vi "Shoot.vi"(10 "User Input":dbl, 11 "Numeric":dbl) -> ()   [LabVIEW 2012]
uses:
  Robot Global Data.vi
panel:
  # "Shoot"
  # "Shooter power ;1. Frount of the 3 point target\n                          2. Frount of 2 point target\n                          3. Key frount of 3 point target \n                          4. User Input"
  # "Input  0 to -1"
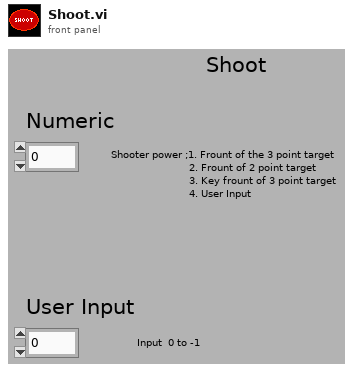
[diagram p1: front panel]
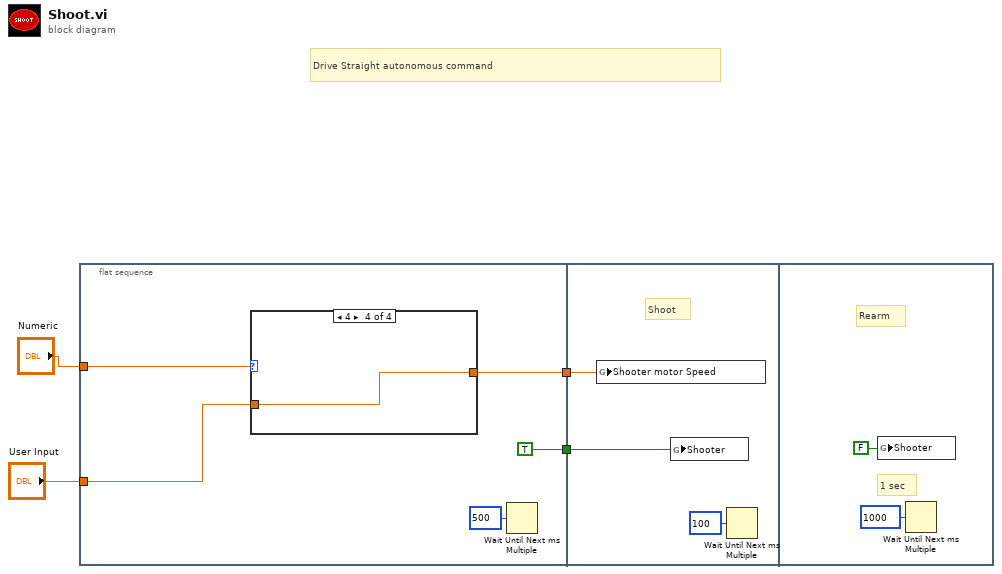
[diagram p0: block diagram]
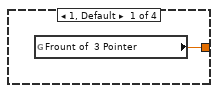
[diagram p2: hidden frame]
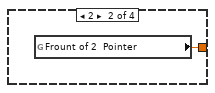
[diagram p3: hidden frame]
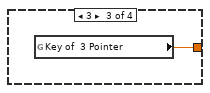
[diagram p4: hidden frame]
diagram:
  # "Drive Straight autonomous command"
  n1 = flat-sequence {
    tunnel: [TRUE] -> w4
    tunnel: "Numeric" -> [w7]
    tunnel: [w6] -> w2
    tunnel: "User Input" -> [w5]
    tunnel: w4 -> [w15]
    tunnel: w2 -> [w14]
    frame #0 {
      n2 = case shown="4" w7 {
        tunnel: [w10 w11 w12 w13] -> w6
        tunnel: w5 -> [_ _ _ w13]
        frame 1, Default {
          n3 = global read "Robot Global Data.vi" "Frount of  3 Pointer"() -> (w10:dbl)
        }
        frame 2 {
          n4 = global read "Robot Global Data.vi" "Frount of 2  Pointer"() -> (w11:dbl)
        }
        frame 3 {
          n5 = global read "Robot Global Data.vi" "Key of  3 Pointer"() -> (w12:dbl)
        }
        frame 4 {
        }
      }
      n6 = Wait Until Next ms Multiple(millisecond multiple=u32 500) -> ()  [unwired: 1 out]
    }
    frame #1 {
      # "Shoot"
      n7 = global write "Robot Global Data.vi" "Shooter motor Speed"(w14) -> ()
      n8 = global write "Robot Global Data.vi" "Shooter"(w15) -> ()
      n9 = Wait Until Next ms Multiple(millisecond multiple=u32 100) -> ()  [unwired: 1 out]
    }
    frame #2 {
      # "1 sec"
      # "Rearm"
      n10 = global write "Robot Global Data.vi" "Shooter"(FALSE ("Shooter")) -> ()
      n11 = Wait Until Next ms Multiple(millisecond multiple=u32 1000) -> ()  [unwired: 1 out]
    }
  }
